vi "CursorPos Read.vi"(4 "error in (no error)":errorcluster, 6 "Container State":T7, 7 "Display State In":T2) -> (0 "error out":errorcluster, 2 "Value":T1, 3 "Display State Out":T2)   [LabVIEW 2015, in "Interactive Graph.xctl"]
uses:
  Interactive Graph.xctl
  <vilib>/_xctls/Container State.ctl
  State.vi
  Persistent.ctl
  Plot.ctl
  EPhys/LV Source/Work Panel VIs/Typedefs/EPhysWork-Label Position.ctl
  Events.ctl
  Selection.ctl
  XRange.ctl
  YScale.ctl
  Cursor.ctl
  <vilib>/Utility/miscctls.llb/LVPointDoubleTypeDef.ctl
  <vilib>/_xctls/XControlSupport.lvlib
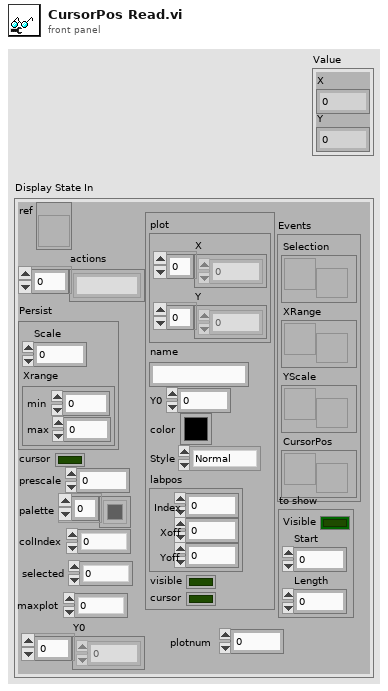
[diagram p1: front panel]
types:
  T1 = typedef "LVPointDoubleTypeDef.ctl" = cluster{"X":dbl, "Y":dbl}
  T2 = typedef "Interactive Graph.xctl/State.vi" = cluster{"ref":refnum<vi>, "actions":string[], "Persist":T3, "cursor":bool, "prescale":dbl, "palette":u32[], "colIndex":i32, "to add":T4, "Events":T6, "selected":i32, "to show":cluster{"Visible":bool, "Start":i32, "Length":i32}, "maxplot":i32, "Y0":dbl[], "plotnum":i32}
  T3 = typedef "Interactive Graph.xctl/Persistent.ctl" = cluster{"Scale":dbl, "Xrange":cluster{"min":dbl, "max":dbl}}
  T4 = typedef "Interactive Graph.xctl/Plot.ctl" = cluster{"plot":cluster{"X":dbl[], "Y":dbl[]}, "name":string, "Y0":dbl, "color":u32, "Style":enum16{"Normal", "Highlight", "Shadow"}, "labpos":T5, "visible":bool, "cursor":bool}
  T5 = typedef "EPhysWork-Label Position.ctl" = cluster{"Index":i32, "Xoff":dbl, "Yoff":dbl}
  T6 = typedef "Interactive Graph.xctl/Events.ctl" = cluster{"Selection":refnum<user-event>, "XRange":refnum<user-event>, "YScale":refnum<user-event>, "CursorPos":refnum<user-event>}
  T7 = typedef "XControlSupport.lvlib/Container State.ctl" = cluster{"Indicator?":bool, "Run Mode?":bool, " Refnum":refnum<vi>}
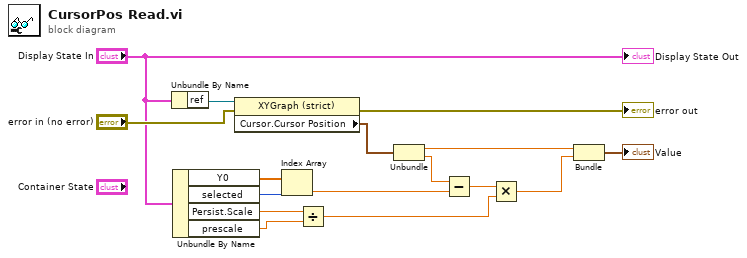
[diagram p0: block diagram]
diagram:
  n1 = Unbundle By Name("Display State In") -> ("ref"=w16:refnum<vi>)
  n2 = Unbundle By Name("Display State In") -> ("Y0"=w8:dbl[], "selected"=w13:i32, "Persist.Scale"=w11:dbl, "prescale"=w1:dbl)
  n3 = property class="XYGraph (strict)"(reference=w16, error in="error in (no error)") -> (error out=→"error out":errorcluster, "Cursor.Cursor Position"=w6:T1)  [unwired: 1 out]
  n4 = Index Array(array=w8, index=w13) -> (element=w7:dbl)
  n5 = Divide(x=w11, y=w1) -> (x/y=w2:dbl)
  n6 = Unbundle(w6) -> ("Cursor X"=w4:dbl, "Cursor Y"=w5:dbl)
  n7 = Subtract(x=w5, y=w7) -> (x-y=w12:dbl)
  n8 = Multiply(x=w12, y=w2) -> (x*y=w10:dbl)
  n9 = Bundle("Cursor X"=w4, w10) -> (→"Value":cluster{"Cursor X":dbl, dbl})  [unwired: 1 in]
  "Display State Out" <- "Display State In"
